vi "parseTemperatureResponse.vi"(8 "error in (no error)":errorcluster, 10 "DynamicFrameParser":refnum<class "DynamicFrameParser.lvclass">, 11 "MTILC in":refnum<class "MTILC.lvclass">) -> (0 "error out":errorcluster, 3 "MTILC out":refnum<class "MTILC.lvclass">)   [LabVIEW 2016, in "RTMTILC.lvlib" / "MTILC.lvclass"]
uses:
  MTILC.lvclass
  Common_RT_Modbus/DynamicFrameParser/DynamicFrameParser.lvclass
  Common_RT_Modbus/DataTypes/ExceptionCodes.ctl
  MTILC.lvclass/MTILC.ctl
  Common_RT_Modbus/RTModbus.lvlib
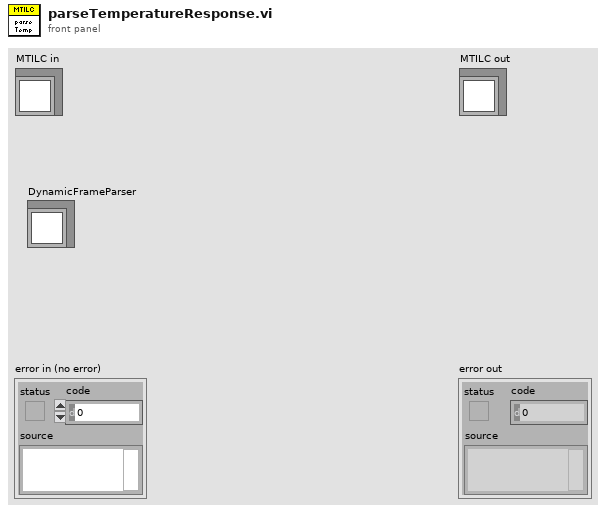
[diagram p1: front panel]
types:
  T1 = typedef "RTModbus.lvlib/ExceptionCodes.ctl" = u16
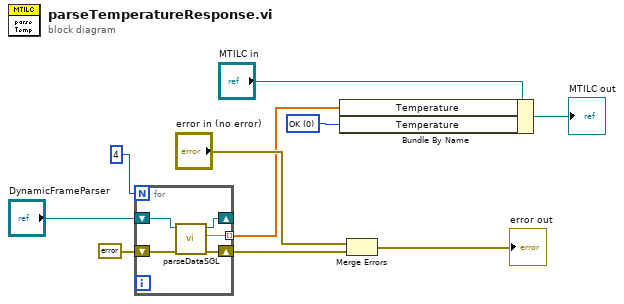
[diagram p0: block diagram]
diagram:
  w6 = T1 0 items=["OK", "IllegalFunction", "IllegalDataAddress", "IllegalDataValue", "SlaveDeviceFailure", "Acknowledge", "SlaveDeviceBusy", "NegativeAcknowledge", "MemoryParityError", "GatewayPathUnavailable", "GatewayTargetDeviceFailedToRespond"] ("MTData.MTResponses.Temperature")
  n1 = for {
    N: 4 -> [_]
    shift-right: [w14] -> w4
    shift-left: errorcluster {"status"=FALSE, "code"=0, "source"=""} ("error out") -> [w13]
    tunnel: [w12] -> w3 mode=indexing
    shift-right: [w11] -> _
    shift-left: "DynamicFrameParser" -> [w15]
    n2 = call "parseDataSGL.vi"("error in (no error)"=w13, "FrameParser in"=w15) -> ("error out"=w14:errorcluster, "Data"=w12:sgl, "FrameParser out"=w11:refnum<class "DynamicFrameParser.lvclass">)  [unwired: 7 in]
  }
  n3 = Bundle By Name(cluster="MTILC in", "Temperature"=w3, "Temperature"=w6) -> (→"MTILC out":refnum<class "MTILC.lvclass">)
  n4 = Merge Errors("error in (no error)", w4) -> (→"error out":errorcluster)
